vi "Project.vi"() -> ()   [LabVIEW 2022 SP3]
uses:
  Control 3.ctl
  Control 1.ctl
  <vilib>/numeric/Random Number (Range) U64.vi
  <vilib>/numeric/sub_Random U32.vi
panel:
  out "Solar pannels manager":T1(tab)
  in  "Slide 26":u8(slide)
  in  "Move to Next State":bool
  out "Discharge State":bool
  out "Charging State":bool
  in  "State selector":bool
  out "summer":picture
  out "spring":picture
  out "winter":picture
  out "Fall":picture
  out "2D Picture":picture
  out "The project is recomended":bool
  out "CRT meter 2":dbl(knob) scale=0.0..10.0
  out "CRT (years) 2":dbl
  in  "Choose your season":enum16{"Winter", "Spring", "Summer", "Fall"}(ring)
  out "IRR":dbl
  in  "Interest Rate %":dbl min=0.0 max=100.0 step=1.0 format="%#_3g"
  in  "Private Generator Availability":bool
  out "Unit Cost":dbl
  out "CRT meter":dbl(knob) scale=0.0..10.0
  out "Unit Cost 2":dbl
  out "Nominal Capacity (kWh)":dbl
  in  "Battery Type":T2(ring)
  out "Min":dbl
  out "Max":dbl
  out "DOD":dbl
  out "Efficiency 2":dbl
  out "Battery capacity (Ah)":dbl
  out "Nominal voltage":dbl
  out "Properties 2":string
  out "Conventional CRT (years)":dbl
  out "Yearly Saving ($)":dbl
  out "Total Installation Cost($)":dbl
  out "BOM($)":dbl
  in  "kWh price ($/kWh)":dbl min=0.0 step=0.01
  out "Numbers of Batteries":dbl
  out "Battery & Inverter Compatibility":string
  out "Number of series (BAT)":dbl
  out "Required Number of Panels":dbl
  in  "Location index":dbl(slide)=5.0 min=4.0 max=8.0 step=1.0 scale=4.0..8.0 scale format="%#_1g"
  out "Reqired Daily Production":dbl
  out "Required Pack Capacity":dbl
  out "Average Consuption":dbl
  in  "Minimum Backup Time (hour)":dbl=6.0 min=6.0 max=24.0 step=1.0 format="%#_2g"
  in  "Monthly Energy Consumption":dbl min=0.0
  in  "Safety factor":dbl=1.25 min=1.25 max=2.0 step=0.01 format="%#_3g"
  out "Total System maximum Draw":dbl
  out "Battery Pack Voltage":dbl
  out "Inverter efficiency":dbl
  out "RMS per phase voltage":dbl
  out "Rated Output Power (kW/PP)":dbl
  out "Triphase":bool
  out "Monophase":bool
  in  "Three-phase-system":bool
  out "Max 2":dbl format="%#_2g"
  in  "Max load ( per phase in kW)":dbl(slide) min=0.0 step=1.0 scale=0.0..50.0 scale format="%#_2g"
  out "INVERTER RECOMANDATION":string
  in  "Solar Panel Type":T3(ring)
  out "Efficiency":dbl
  out "Cost per panel":dbl
  out "Rated power":dbl
  out "Properties":string
  in  "Simulate Charging":bool
  in  "LOAD":dbl(slide) min=0.0 max=99.0 step=1.0 scale=0.0..100.0
  in  "Next State":bool
  in  "Seasons effect":bool
  in  "Light Intensity/ Irradiance, W/m^2:":dbl(knob)=600.0 min=0.0 max=2000.0 step=1.0 scale=0.0..1200.0
  in  "BATTERY CAPACITY (OV)":bool
  in  "Current Batterie %":dbl
  out "Batteries Power":dbl(knob) scale=0.0..10.0
  out "I_E":dbl
  out "Charge_Time":dbl
  out "BAT_DOD":dbl
  out "BAT_E":dbl
  in  "BATTERY PACK CAPACITY (OV)":dbl
  out "Array Rated power":dbl
  in  "Season":T4
  out "Solar Panel instantaneous P":dbl(knob) scale=0.0..10.0
  out "Load -Usage":dbl(knob) scale=0.0..2.0
  out "Private Generator 2":dbl(knob) scale=0.0..3.0
  out "Battery Level 2":dbl(slide) scale=0.0..100.0
  in  "Next State":bool
  in  "Start Simulation":bool
  in  "Load override":bool
  out "Batteries Power 2":dbl(knob) scale=0.0..10.0
  out "Load 3":dbl(knob) scale=0.0..5.0
  out "Private-Generatot 3":dbl(knob) scale=0.0..3.0
  out "Battery Level 3":dbl(slide) scale=0.0..100.0
  in  "Load override\n( per phase in kW)":dbl(slide) scale=0.0..10.0
  out "Total_Discharge_Time":dbl
  in  "Season 2":T4
  out "BAT_DOD 2":dbl
  out "I_E 2":dbl
  in  "Go back to Initialize":bool
  out "MESSAGE":string
  in  "Slide 25":u8(slide)
  # "SOLAR PANEL DESIGN"
  # "MADE BY"
  # "ELIAS ISHAK \nGEORGE YAMMINE \nELIE NAJM \nELIAS RIZK \nJACQUES MKHAYEL \nCHRISTOPHE RECHDAN"
  # "Economy"
  # "bekaaa"
  # "north ,south"
  # "beirut"
  # "matn"
  # "Thank You For Choosing us"
  # "About us :"
  # "About us:\nkindly check our website @ \nsolarpannelsmanager.com"
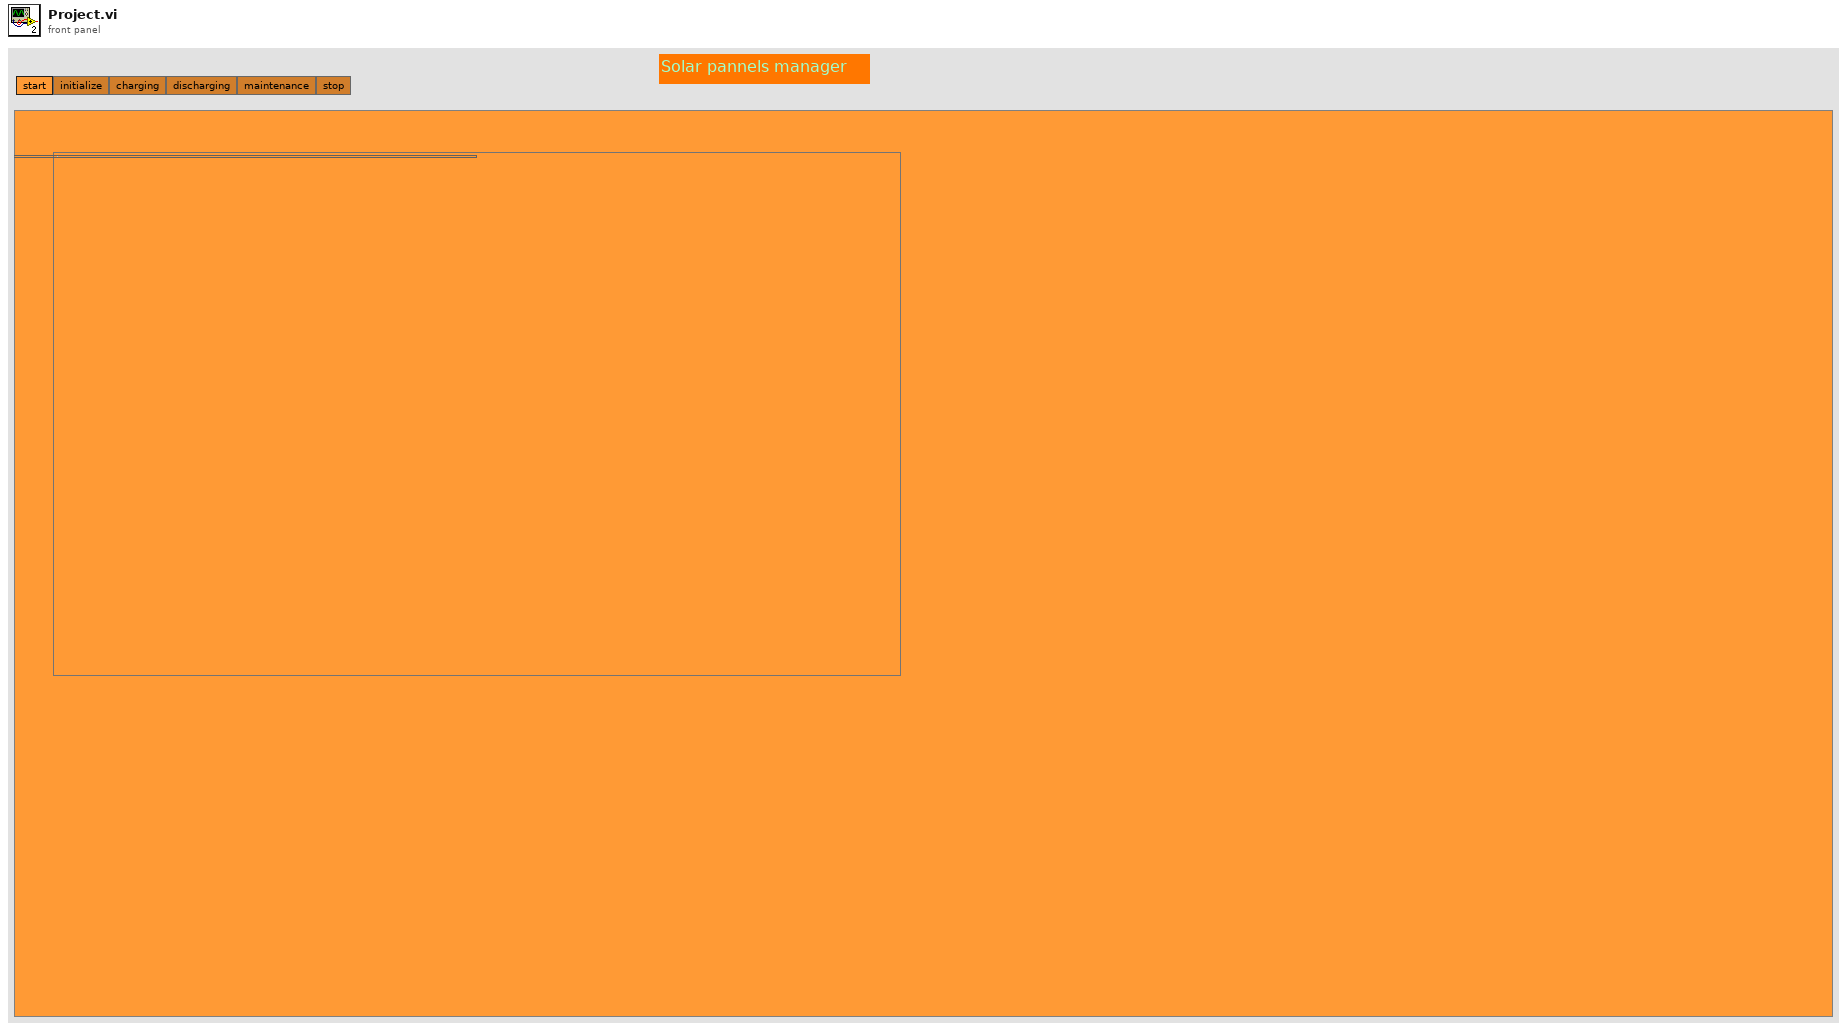
[diagram p1: front panel]
types:
  T1 = enum32{"start", "initialize", "charging", "discharging", "maintenance", "stop"}
  T2 = enum16{"Lead acid flood", "Lead acid sealed", "Lead acid agm", "Li-ion", "Li-FePO4", "Li-po"}
  T3 = enum16{"Monocrinstalin-biface", "Monocristalin", "Polycristalin", "Amorph"}
  T4 = typedef "Control 3.ctl" = enum16{"Fall", "Spring", "Winter", "Summer"}
  T5 = typedef "Control 1.ctl" = enum16{"start state ", "Initialize State", "charging state ", "discharging state ", "maintenance ", "Stop State"}
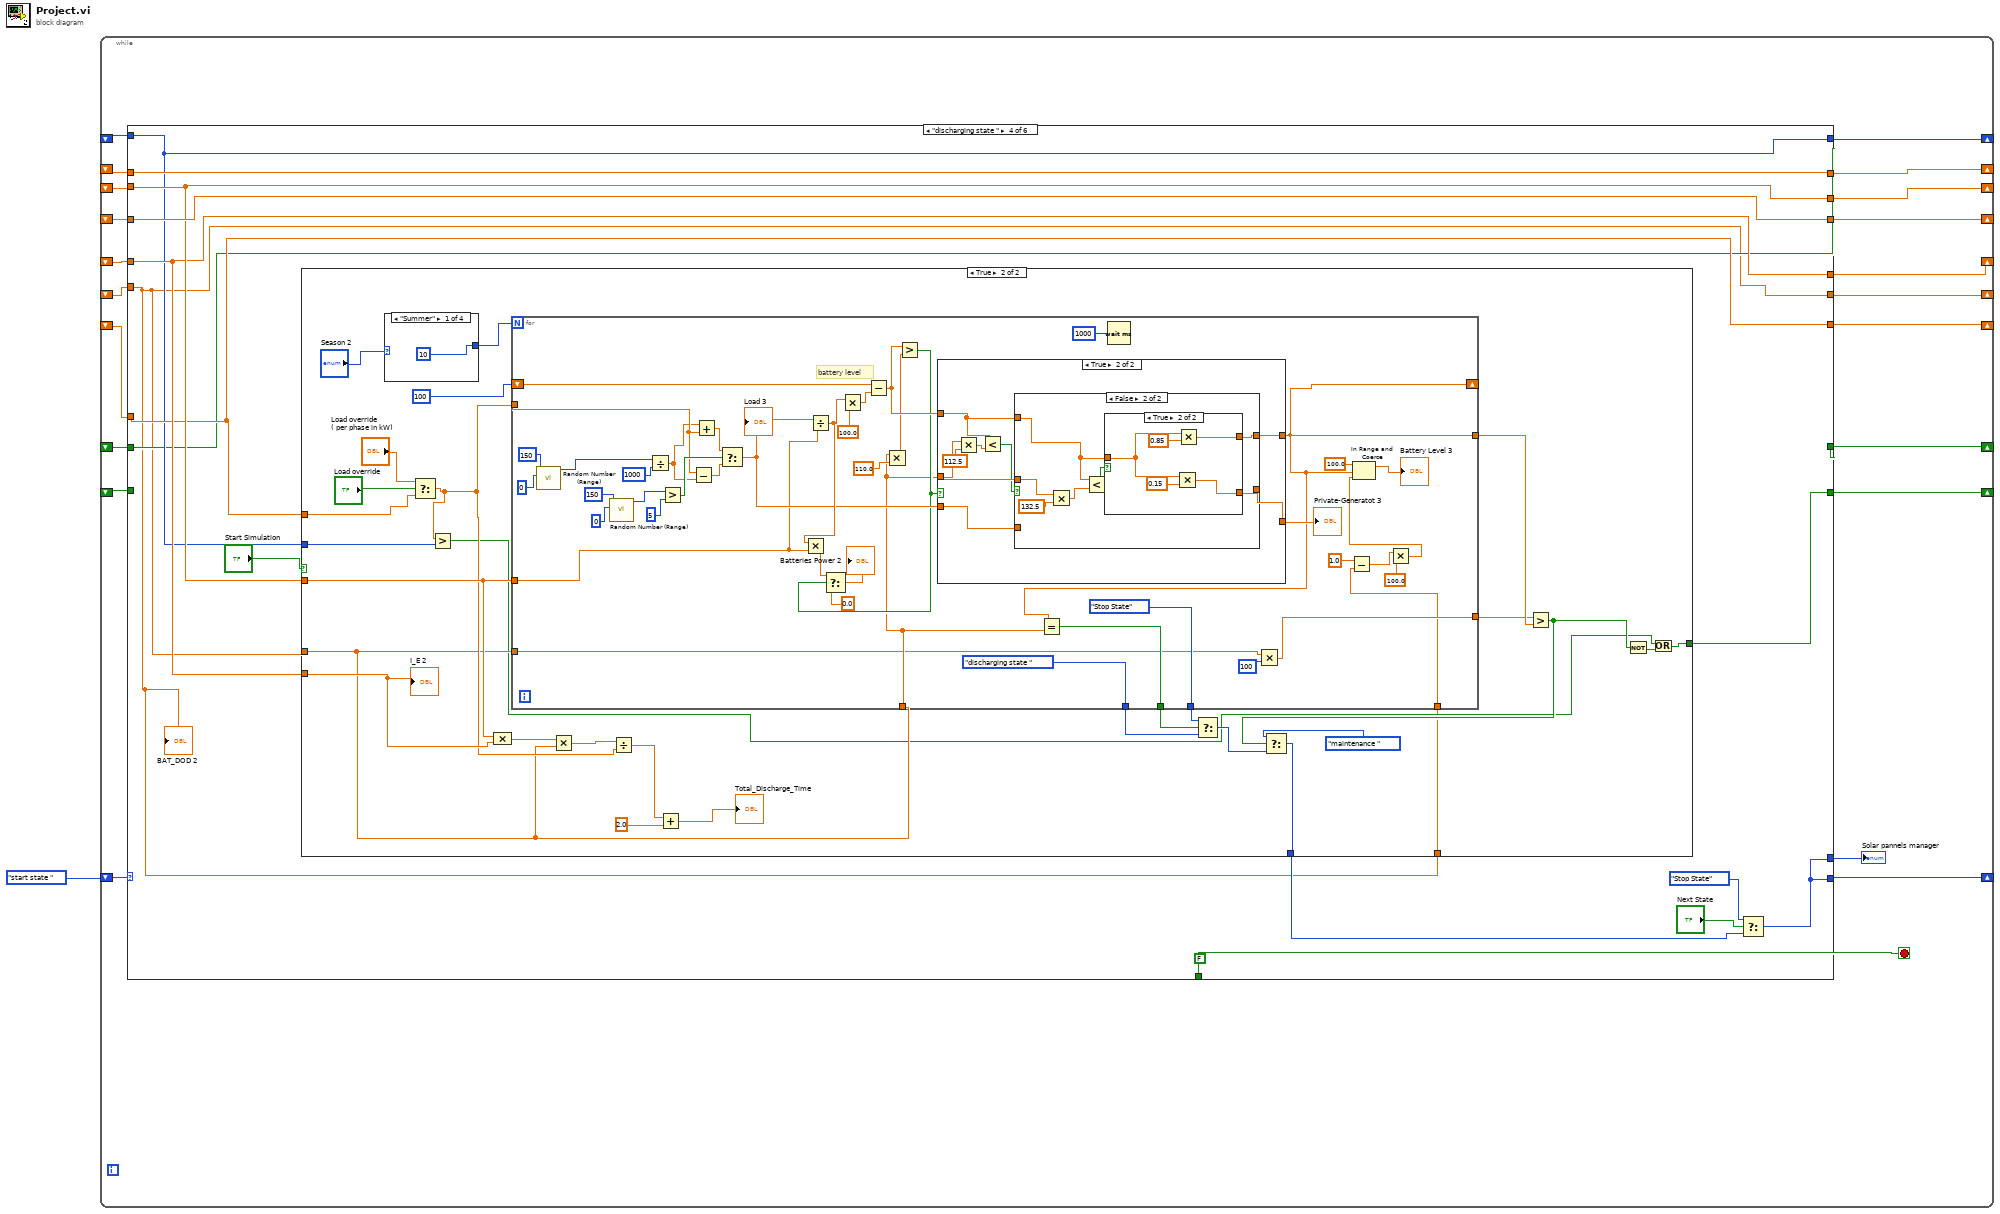
[diagram p0: block diagram]
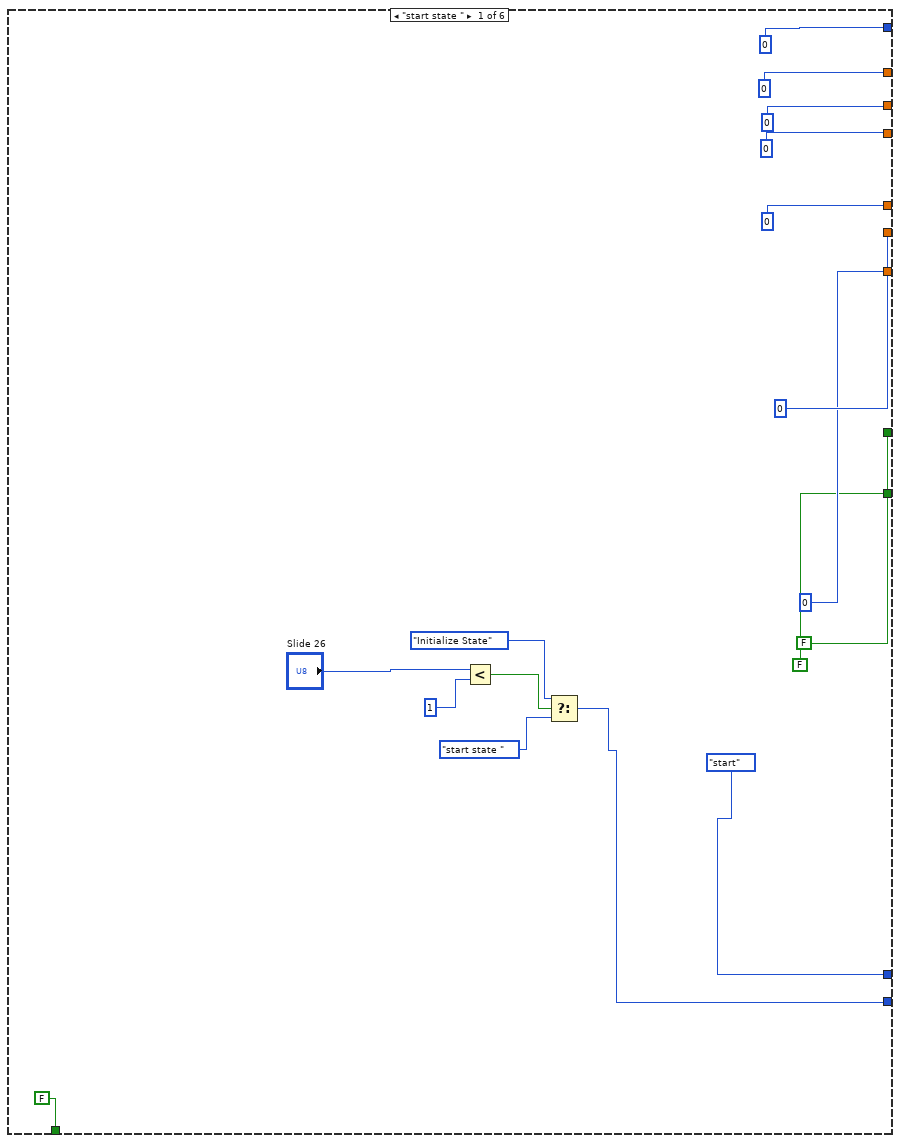
[diagram p2: hidden frame]
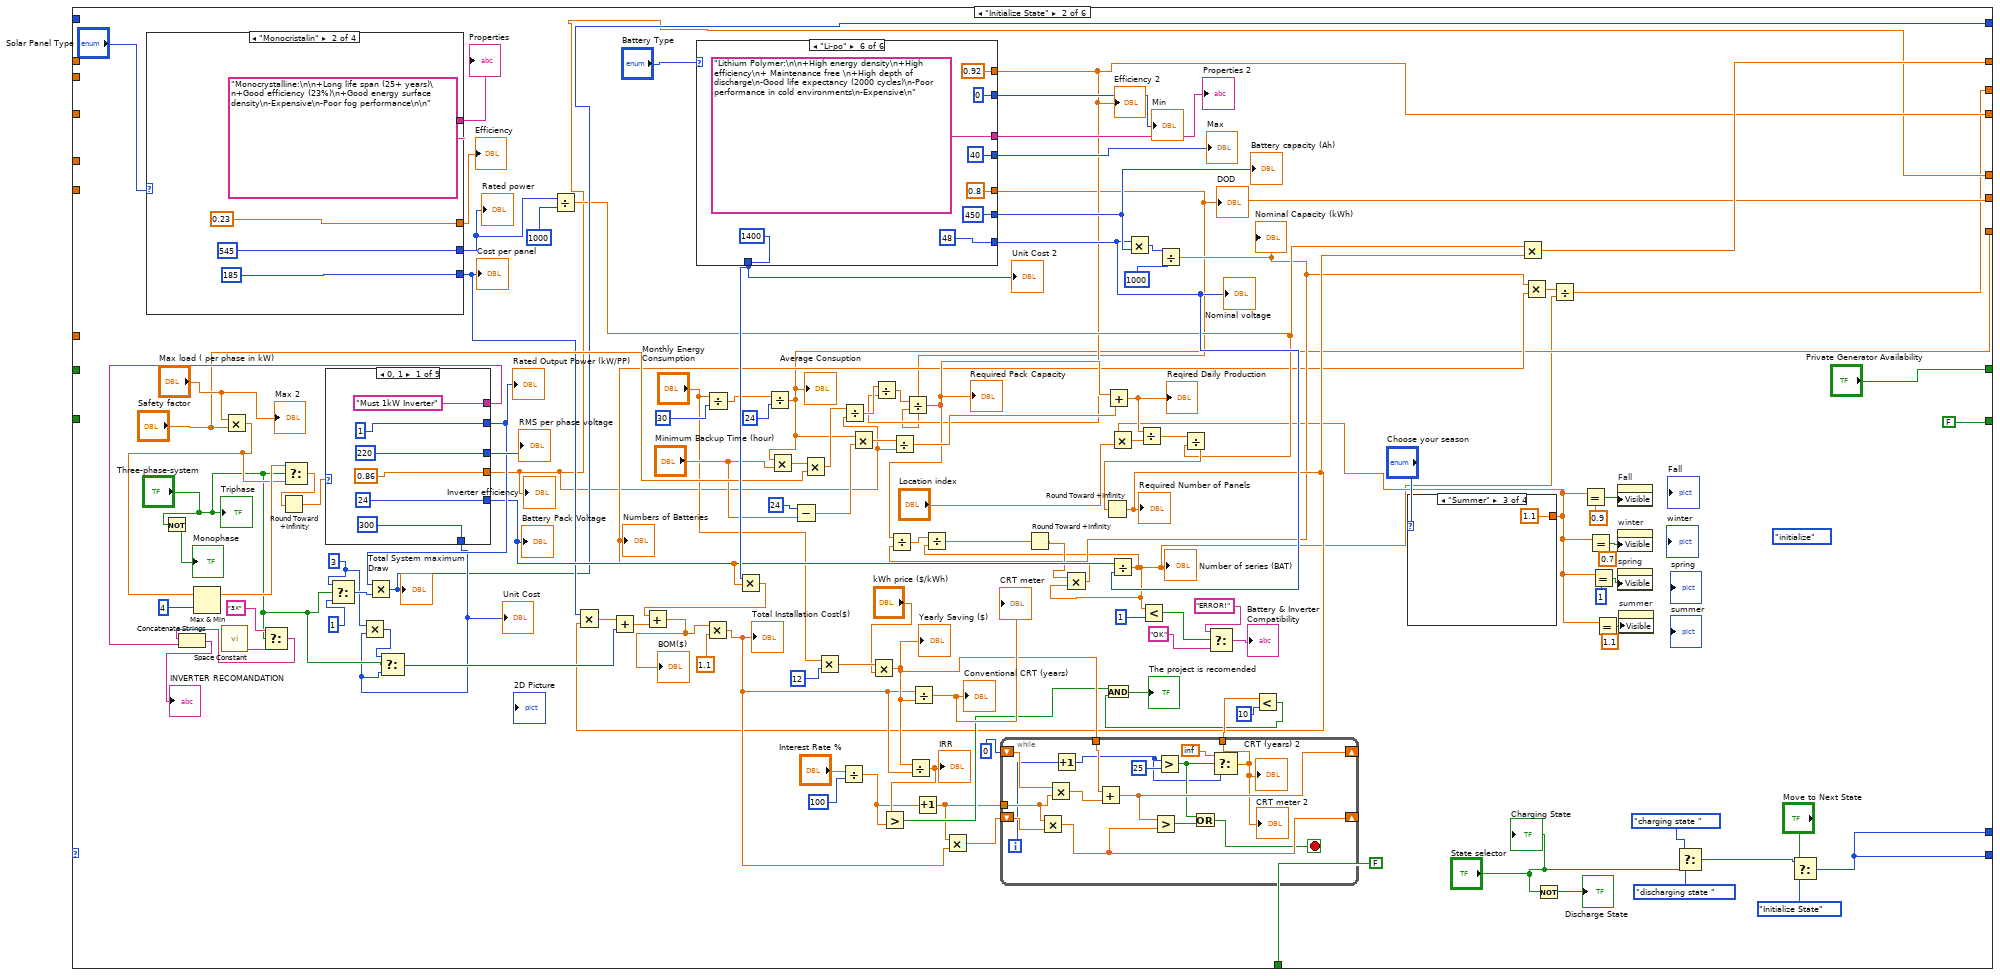
[diagram p3: hidden frame]
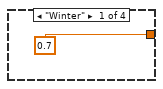
[diagram p4: hidden frame]
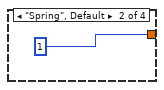
[diagram p5: hidden frame]
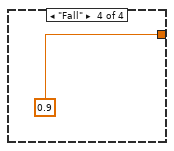
[diagram p6: hidden frame]
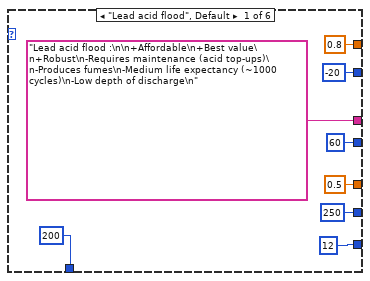
[diagram p7: hidden frame]
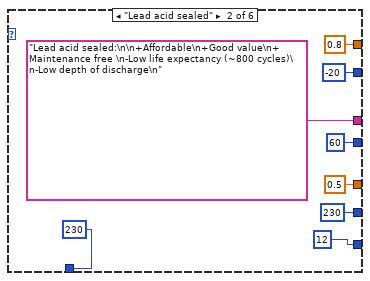
[diagram p8: hidden frame]
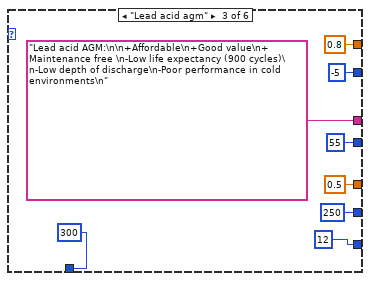
[diagram p9: hidden frame]
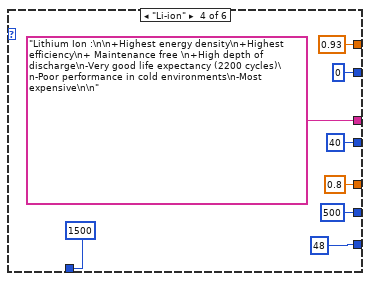
[diagram p10: hidden frame]
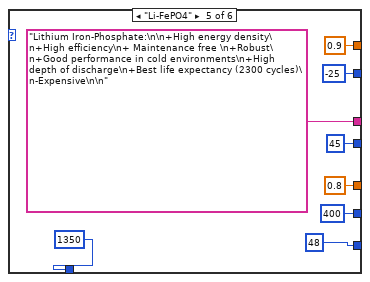
[diagram p11: hidden frame]
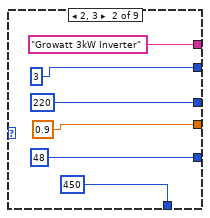
[diagram p12: hidden frame]
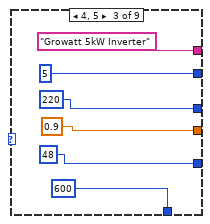
[diagram p13: hidden frame]
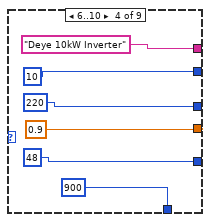
[diagram p14: hidden frame]
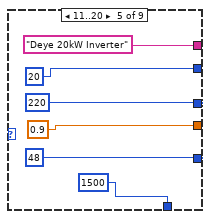
[diagram p15: hidden frame]
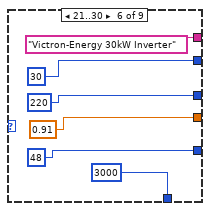
[diagram p16: hidden frame]
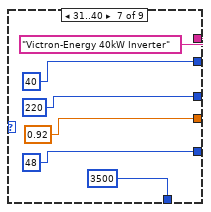
[diagram p17: hidden frame]
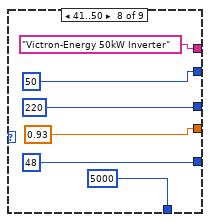
[diagram p18: hidden frame]
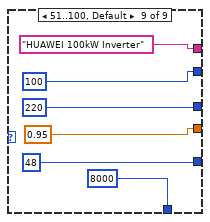
[diagram p19: hidden frame]
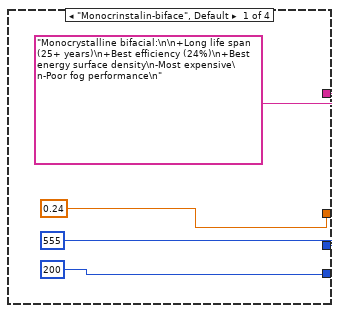
[diagram p20: hidden frame]
diagram:
  n1 = while {
    shift-right: [w22] -> _
    shift-left: Control_1."start state " ("Status") -> [w23]
    shift-right: [w19] -> _
    shift-left: _ -> [w18]
    shift-right: [w17] -> _
    shift-left: _ -> [w16]
    shift-right: [w14] -> _
    shift-left: _ -> [w15]
    shift-right: [w12] -> _
    shift-left: _ -> [w13]
    shift-right: [w10] -> _
    shift-left: _ -> [w11]
    shift-right: [w8] -> _
    shift-left: _ -> [w9]
    shift-right: [w7] -> _
    shift-left: _ -> [w6]
    shift-right: [w5] -> _
    shift-left: _ -> [w4]
    shift-right: [w2] -> _
    shift-left: _ -> [w3]
    stop <- w21 stop-if-true
    n2 = case shown="\"discharging state \"" w23 {
      tunnel: [w29 w48 w305 w434 w554 w576] -> w22
      tunnel: [FALSE FALSE FALSE FALSE FALSE TRUE] -> w21
      tunnel: [T1."start" ("Tab Control") w48 w305 w434 w554 T1."stop" ("Tab Control")] -> w20
      tunnel: [0 w58 w312 w440 w574 0] -> w19
      tunnel: w18 -> [_ _ w312 w440 w574 _]
      tunnel: [0 w55 w319 w445 w573 0] -> w17
      tunnel: w16 -> [_ _ w319 w445 w573 _]
      tunnel: w15 -> [_ _ w318 w443 w572 _]
      tunnel: [0 w41 w318 w443 w572 0] -> w14
      tunnel: w13 -> [_ _ w317 w444 w571 _]
      tunnel: [0 w52 w317 w444 w571 0] -> w12
      tunnel: w11 -> [_ _ w316 w442 w570 _]
      tunnel: [0 w51 w316 w442 w570 0] -> w10
      tunnel: w9 -> [_ _ w315 w432 w569 _]
      tunnel: [0 w50 w315 w432 w569 0] -> w8
      tunnel: [0 w47 w310 w441 w568 0] -> w7
      tunnel: w6 -> [_ _ w310 w441 w568 _]
      tunnel: [FALSE "Private Generator Availability" w309 w433 w567 FALSE] -> w5
      tunnel: w4 -> [_ _ w309 w433 w567 _]
      tunnel: [FALSE FALSE w308 w439 w564 FALSE] -> w2
      tunnel: w3 -> [_ _ _ _ w564 _]
      frame "start state " {
        n3 = Less?(x="Slide 26", y=1) -> (x < y?=w25:bool)
        n4 = Select(t=Control_1."Initialize State" ("Status"), s=w25, f=Control_1."start state " ("Status")) -> (s? t:f=w29:T5)
      }
      frame "Initialize State" {
        w113 = 3
        (unwired) T1."initialize" ("Tab Control")
        n5 = case shown="\"Monocristalin\"" "Solar Panel Type" {
          tunnel: ["Monocrystalline bifacial:\n\n+Long life span (25+ years)\n+Best efficiency (24%)\n+Best energy surface density\n-Most expensive\n-Poor fog performance\n" "Monocrystalline:\n\n+Long life span (25+ years)\n+Good efficiency (23%)\n+Good energy surface density\n-Expensive\n-Poor fog performance\n\n" "Polycrystalline:\n\n+Good life span (15+ years)\n+Offers the best value\n+Good efficiency (20%)\n-Poor fog performance\n\n" "Amorphous:\n\n+Acceptable life span (10+ years)\n+Affordable\n+Good fog performance \n-Low efficiency (10%)\n\n"] -> w160
          tunnel: [555 545 500 200] -> w98
          tunnel: [0.24 0.23 0.2 0.1] -> w159
          tunnel: [200 185 160 100] -> w96
          frame "Monocrinstalin-biface", Default {
          }
          frame "Monocristalin" {
          }
          frame "Polycristalin" {
          }
          frame "Amorph" {
          }
        }
        "Properties" <- w160
        "Rated power" <- w98
        "Cost per panel" <- w96
        "Efficiency" <- w159
        n6 = Not(x="Three-phase-system") -> (.not. x?=→"Monophase":bool)
        n7 = call <vilib>:"Space Constant.vi"() -> ("String"=w153:string)
        n8 = Multiply(x="Max load ( per phase in kW)", y="Safety factor") -> (x*y=w147:dbl)
        n9 = Max & Min(x=w147, y=4) -> (max(x,y)=w155:dbl)  [unwired: 1 out]
        n10 = Select(t="3X", s="Three-phase-system", f=w153) -> (s? t:f=w152:string)
        n11 = Select(t=w155, s="Three-phase-system", f=w147) -> (s? t:f=w105:dbl)
        n12 = Round Toward +Infinity(x=w105) -> (ceil(x): smallest int >= x=w104:dbl)
        n13 = case shown="0, 1" w104 {
          tunnel: ["Must 1kW Inverter" "Growatt 3kW Inverter" "Growatt 5kW Inverter" "Deye 10kW Inverter" "Deye 20kW Inverter" "Victron-Energy 30kW Inverter" "Victron-Energy 40kW Inverter" "Victron-Energy 50kW Inverter" "HUAWEI 100kW Inverter"] -> w151
          tunnel: [1 3 5 10 20 30 40 50 100] -> w145
          tunnel: [220 220 220 220 220 220 220 220 220] -> w149
          tunnel: [0.86 0.9 0.9 0.9 0.9 0.91 0.92 0.93 0.95] -> w51
          tunnel: [24 48 48 48 48 48 48 48 48] -> w127
          tunnel: [300 450 600 900 1500 3000 3500 5000 8000] -> w92
          frame 0, 1 {
          }
          frame 2, 3 {
          }
          frame 4, 5 {
          }
          frame 6..10 {
          }
          frame 11..20 {
          }
          frame 21..30 {
          }
          frame 31..40 {
          }
          frame 41..50 {
          }
          frame 51..100, Default {
          }
        }
        "Rated Output Power (kW/PP)" <- w145
        "RMS per phase voltage" <- w149
        "Inverter efficiency" <- w51
        "Battery Pack Voltage" <- w127
        "Unit Cost" <- w92
        n14 = Concatenate Strings(w152, w151) -> (→"INVERTER RECOMANDATION":string)
        n15 = Select(t=w113, s="Three-phase-system", f=1) -> (s? t:f=w146:i32)
        n16 = Multiply(x=w113, y=w92) -> (x*y=w114:i32)
        n17 = Multiply(x=w145, y=w146) -> (x*y=w58:i32)
        "Total System maximum Draw" <- w58
        n18 = Select(t=w114, s="Three-phase-system", f=w92) -> (s? t:f=w115:i32)
        n19 = Divide(x=w98, y=1000) -> (x/y=w57:dbl)
        n20 = case shown="\"Li-po\"" "Battery Type" {
          tunnel: ["Lead acid flood :\n\n+Affordable\n+Best value\n+Robust\n-Requires maintenance (acid top-ups)\n-Produces fumes\n-Medium life expectancy (~1000 cycles)\n-Low depth of discharge\n" "Lead acid sealed:\n\n+Affordable\n+Good value\n+ Maintenance free \n-Low life expectancy (~800 cycles)\n-Low depth of discharge\n" "Lead acid AGM:\n\n+Affordable\n+Good value\n+ Maintenance free \n-Low life expectancy (900 cycles)\n-Low depth of discharge\n-Poor performance in cold environments\n" "Lithium Ion :\n\n+Highest energy density\n+Highest efficiency\n+ Maintenance free \n+High depth of discharge\n-Very good life expectancy (2200 cycles)\n-Poor performance in cold environments\n-Most expensive\n\n" "Lithium Iron-Phosphate:\n\n+High energy density\n+High efficiency\n+ Maintenance free \n+Robust\n+Good performance in cold environments\n+High depth of discharge\n+Best life expectancy (2300 cycles)\n-Expensive\n\n" "Lithium Polymer:\n\n+High energy density\n+High efficiency\n+ Maintenance free \n+High depth of discharge\n-Good life expectancy (2000 cycles)\n-Poor performance in cold environments\n-Expensive\n"] -> w103
          tunnel: [0.5 0.5 0.5 0.8 0.8 0.8] -> w50
          tunnel: [0.8 0.8 0.8 0.93 0.9 0.92] -> w52
          tunnel: [12 12 12 48 48 48] -> w82
          tunnel: [250 230 250 500 400 450] -> w99
          tunnel: [60 60 55 40 45 40] -> w102
          tunnel: [-20 -20 -5 0 -25 0] -> w101
          tunnel: [200 230 300 1500 1350 1400] -> w161
          frame "Lead acid flood", Default {
          }
          frame "Lead acid sealed" {
          }
          frame "Lead acid agm" {
          }
          frame "Li-ion" {
          }
          frame "Li-FePO4" {
          }
          frame "Li-po" {
          }
        }
        "Properties 2" <- w103
        "Nominal voltage" <- w82
        "Battery capacity (Ah)" <- w99
        "Efficiency 2" <- w52
        "DOD" <- w50
        "Max" <- w102
        "Min" <- w101
        "Unit Cost 2" <- w161
        n21 = Divide(x="Monthly Energy Consumption", y=30) -> (x/y=w138:dbl)
        n22 = Divide(x=w138, y=24) -> (x/y=w47:dbl)
        "Average Consuption" <- w47
        n23 = Multiply(x=w47, y="Minimum Backup Time (hour)") -> (x*y=w140:dbl)
        n24 = Subtract(x=24, y="Minimum Backup Time (hour)") -> (x-y=w133:dbl)
        n25 = Multiply(x=w140, y="Safety factor") -> (x*y=w135:dbl)
        n26 = Multiply(x="Monthly Energy Consumption", y=12) -> (x*y=w107:dbl)
        n27 = Divide(x="Interest Rate %", y=100) -> (x/y=w87:dbl)
        n28 = Divide(x=w135, y=w51) -> (x/y=w136:dbl)
        n29 = Multiply(x=w47, y=w133) -> (x*y=w137:dbl)
        n30 = Multiply(x=w107, y="kWh price ($/kWh)") -> (x*y=w86:dbl)
        "Yearly Saving ($)" <- w86
        n31 = Divide(x=w136, y=w52) -> (x/y=w141:dbl)
        n32 = Divide(x=w137, y=w51) -> (x/y=w134:dbl)
        n33 = Divide(x=w141, y=w50) -> (x/y=w121:dbl)
        "Required Pack Capacity" <- w121
        n34 = Increment(x=w87) -> (x+1=w75:dbl)
        n35 = Add(x=w121, y=w134) -> (x+y=w130:dbl)
        "Reqired Daily Production" <- w130
        n36 = Divide(x=w127, y=w82) -> (x/y=w42:dbl)
        "Number of series (BAT)" <- w42
        n37 = Multiply(x=w82, y=w99) -> (x*y=w94:i32)
        n38 = Less?(x=w42, y=1) -> (x < y?=w125:bool)
        n39 = Divide(x=w94, y=1000) -> (x/y=w54:dbl)
        "Nominal Capacity (kWh)" <- w54
        n40 = Divide(x=w121, y=w54) -> (x/y=w120:dbl)
        n41 = Divide(x=w120, y=w42) -> (x/y=w119:dbl)
        n42 = Round Toward +Infinity(x=w119) -> (ceil(x): smallest int >= x=w118:dbl)
        n43 = Multiply(x=w118, y=w42) -> (x*y=w53:dbl)
        "Numbers of Batteries" <- w53
        n44 = Multiply(x=w161, y=w53) -> (x*y=w111:dbl)
        n45 = Select(t="ERROR!", s=w125, f="OK") -> (s? t:f=→"Battery & Inverter Compatibility":string)
        n46 = case shown="\"Summer\"" "Choose your season" {
          tunnel: [0.7 1 1.1 0.9] -> w44
          frame "Winter" {
          }
          frame "Spring", Default {
          }
          frame "Summer" {
          }
          frame "Fall" {
          }
        }
        n47 = Multiply(x=w44, y="Location index") -> (x*y=w84:dbl)
        n48 = Divide(x=w130, y=w84) -> (x/y=w129:dbl)
        n49 = Divide(x=w129, y=w57) -> (x/y=w128:dbl)
        n50 = Round Toward +Infinity(x=w128) -> (ceil(x): smallest int >= x=w56:dbl)
        "Required Number of Panels" <- w56
        n51 = Multiply(x=w96, y=w56) -> (x*y=w117:dbl)
        n52 = Add(x=w117, y=w115) -> (x+y=w112:dbl)
        n53 = Add(x=w111, y=w112) -> (x+y=w109:dbl)
        "BOM($)" <- w109
        n54 = Multiply(x=w109, y=1.1) -> (x*y=w74:dbl)
        "Total Installation Cost($)" <- w74
        n55 = Divide(x=w86, y=w74) -> (x/y=w88:dbl)
        "IRR" <- w88
        n56 = Greater?(x=w88, y=w87) -> (0:w76:bool)
        n57 = Divide(x=w74, y=w86) -> (x/y=→"Conventional CRT (years)" →"CRT meter":dbl)
        n58 = Multiply(x=w75, y=w74) -> (x*y=w73:dbl)
        n59 = while {
          shift-right: [w180] -> _
          shift-left: 0 -> [w178]
          tunnel: w86 -> [w177]
          shift-right: [w179] -> _
          shift-left: w73 -> [w181]
          tunnel: [w170] -> w78
          tunnel: w75 -> [w169]
          i -> [w167]
          stop <- w172 stop-if-true
          n60 = Multiply(x=w169, y=w181) -> (x*y=w179:dbl)
          n61 = Multiply(x=w178, y=w169) -> (x*y=w176:dbl)
          n62 = Increment(x=w167) -> (x+1=w168:i32)
          n63 = Add(x=w177, y=w176) -> (x+y=w180:dbl)
          n64 = Greater?(x=w180, y=w179) -> (0:w173:bool)
          n65 = Greater?(x=w168, y=25) -> (0:w171:bool)
          n66 = Or(x=w171, y=w173) -> (x .or. y?=w172:bool)
          n67 = Select(t=inf, s=w171, f=w168) -> (s? t:f=w170:dbl)
          "CRT (years) 2" <- w170
          "CRT meter 2" <- w170
        }
        n68 = Less?(x=w78, y=10) -> (x < y?=w77:bool)
        n69 = And(x=w76, y=w77) -> (x .and. y?=→"The project is recomended":bool)
        n70 = Multiply(x=w57, y=w56) -> (x*y=w55:dbl)
        n71 = Multiply(x=w54, y=w53) -> (x*y=w43:dbl)
        n72 = Not(x="State selector") -> (.not. x?=→"Discharge State":bool)
        n73 = Divide(x=w43, y=w42) -> (x/y=w41:dbl)
        n74 = Equal?(x=w44, y=0.9) -> (x = y?=w71:bool)
        n75 = Equal?(x=w44, y=0.7) -> (x = y?=w69:bool)
        n76 = Equal?(x=w44, y=1) -> (x = y?=w67:bool)
        n77 = Equal?(x=w44, y=1.1) -> (x = y?=w65:bool)
        n78 = property on="Fall" class="Pict"("Visible"=w71) -> ()  [unwired: 2 in, 2 out]
        n79 = property on="winter" class="Pict"("Visible"=w69) -> ()  [unwired: 2 in, 2 out]
        n80 = property on="spring" class="Pict"("Visible"=w67) -> ()  [unwired: 2 in, 2 out]
        n81 = property on="summer" class="Pict"("Visible"=w65) -> ()  [unwired: 2 in, 2 out]
        n82 = Select(t=Control_1."charging state " ("Status"), s="State selector", f=Control_1."discharging state " ("Status")) -> (s? t:f=w62:T5)
        n83 = Select(t=w62, s="Move to Next State", f=Control_1."Initialize State" ("Status")) -> (s? t:f=w48:T5)
        "Max 2" <- "Max load ( per phase in kW)"
        "Triphase" <- "Three-phase-system"
        "Charging State" <- "State selector"
      }
      frame "charging state " {
        w306 = Control_1."maintenance " ("Status")
        n84 = Greater?(x="LOAD", y=w312) -> (0:w302:bool)
        n85 = case shown="True" "Simulate Charging" {
          tunnel: "LOAD" -> [w338 _]
          tunnel: w319 -> [w321 _]
          tunnel: w318 -> [w334 _]
          tunnel: w317 -> [w333 _]
          tunnel: w316 -> [w332 _]
          tunnel: w315 -> [w331 _]
          tunnel: [TRUE FALSE] -> w308
          tunnel: w302 -> [w324 _]
          tunnel: [w323 Control_1."charging state " ("Status")] -> w301
          frame True {
            n86 = Divide(x="Light Intensity/ Irradiance, W/m^2:", y=1000) -> (x/y=w328:dbl)
            n87 = Select(t=w334, s="BATTERY CAPACITY (OV)", f="BATTERY PACK CAPACITY (OV)") -> (s? t:f=w336:dbl)
            n88 = Multiply(x=w328, y=w321) -> (x*y=w327:dbl)
            n89 = Compound Arithmetic op=MULTIPLY(w321, w333, w332, w331) -> (w345:dbl)
            n90 = Divide(x=w336, y=w345) -> (x/y=→"Charge_Time":dbl)
            n91 = case shown="\"Fall\"" "Season" {
              tunnel: w321 -> [w407 w414 w421 w428]
              tunnel: [14 11 10 13] -> w344
              tunnel: [w404 w412 w418 w426] -> w343
              tunnel: w327 -> [w403 w409 w417 w423]
              tunnel: "Seasons effect" -> [w405 w411 w419 w425]
              frame "Summer" {
                n92 = Multiply(x=w407, y=1.0) -> (x*y=w402:dbl)
                n93 = Select(t=w403, s=w405, f=w402) -> (s? t:f=w404:dbl)
              }
              frame "Fall" {
                n94 = Multiply(x=w414, y=0.5) -> (x*y=w410:dbl)
                n95 = Select(t=w409, s=w411, f=w410) -> (s? t:f=w412:dbl)
              }
              frame "Winter" {
                n96 = Multiply(x=w421, y=0.35) -> (x*y=w416:dbl)
                n97 = Select(t=w417, s=w419, f=w416) -> (s? t:f=w418:dbl)
              }
              frame "Spring" {
                n98 = Multiply(x=w428, y=0.7) -> (x*y=w424:dbl)
                n99 = Select(t=w423, s=w425, f=w424) -> (s? t:f=w426:dbl)
              }
            }
            n100 = for {
              N: w344 -> [_]
              tunnel: w343 -> [w360]
              tunnel: w338 -> [w382]
              tunnel: w336 -> [w347]
              shift-right: [w348] -> _
              shift-left: "Current Batterie %" -> [w373]
              n101 = call-poly <vilib>:"Random Number (Range).vi"("lower bound (0)"=u64 0, "upper bound (100)"=u64 10) -> ("number"=w367:u64)  [unwired: 9 in]
              n102 = call-poly <vilib>:"Random Number (Range).vi"("lower bound (0)"=u64 0, "upper bound (100)"=u64 150) -> ("number"=w362:u64)  [unwired: 9 in]
              n103 = call-poly <vilib>:"Random Number (Range).vi"("lower bound (0)"=u64 0, "upper bound (100)"=u64 100) -> ("number"=w389:u64)  [unwired: 9 in]
              n104 = call-poly <vilib>:"Random Number (Range).vi"("lower bound (0)"=u64 0, "upper bound (100)"=u64 10) -> ("number"=w393:u64)  [unwired: 9 in]
              n105 = Divide(x=w362, y=1000.0) -> (x/y=w361:dbl)
              n106 = Greater?(x=w367, y=u64 5) -> (0:w365:bool)
              n107 = Divide(x=w389, y=u64 1000) -> (x/y=w381:dbl)
              n108 = Greater?(x=w393, y=u64 5) -> (0:w392:bool)
              n109 = Add(x=w361, y=w360) -> (x+y=w364:dbl)
              n110 = Subtract(x=w360, y=w361) -> (x-y=w363:dbl)
              n111 = Subtract(x=w382, y=w381) -> (x-y=w390:dbl)
              n112 = Add(x=w381, y=w382) -> (x+y=w391:dbl)
              n113 = Select(t=w364, s=w365, f=w363) -> (s? t:f=w355:dbl)
              "Solar Panel instantaneous P" <- w355
              n114 = Select(t=w391, s=w392, f=w390) -> (s? t:f=w375:dbl)
              "Load -Usage" <- w375
              n115 = Divide(x=w355, y=4.0) -> (x/y=w374:dbl)
              n116 = Subtract(x=w355, y=w375) -> (x-y=w401:dbl)
              n117 = Divide(x=w374, y=w347) -> (x/y=w359:dbl)
              n118 = Divide(x=w401, y=w347) -> (x/y=w358:dbl)
              n119 = Multiply(x=0.75, y=w355) -> (x*y=w356:dbl)
              n120 = Subtract(x=w375, y=w356) -> (x-y=w379:dbl)
              n121 = Multiply(x=w358, y=100.0) -> (x*y=w398:dbl)
              n122 = In Range and Coerce(upper limit=100.0, x=w379, lower limit=0.0) -> (coerced(x)=w352:dbl)  [unwired: 1 out]
              n123 = Less?(x=w398, y=0.0) -> (x < y?=w351:bool)
              n124 = Select(t=w359, s=w351, f=w358) -> (s? t:f=w357:dbl)
              n125 = Select(t=w352, s=w351, f=0.0) -> (s? t:f=w349:dbl)
              "Private Generator 2" <- w349
              n126 = Multiply(x=w347, y=w357) -> (x*y=→"Batteries Power":dbl)
              n127 = Add(x=w349, y=w373) -> (x+y=w396:dbl)
              n128 = Add(x=w373, y=w398) -> (x+y=w395:dbl)
              n129 = Select(t=w396, s=w351, f=w395) -> (s? t:f=w348:dbl)
              n130 = In Range and Coerce(upper limit=100.0, x=w348, lower limit=0.0) -> (coerced(x)=→"Battery Level 2":dbl)  [unwired: 1 out]
              n131 = Wait (ms)(milliseconds to wait=u32 1000) -> ()  [unwired: 1 out]
            }
            n132 = Select(t=Control_1."maintenance " ("Status"), s=w324, f=Control_1."discharging state " ("Status")) -> (s? t:f=w323:T5)
            "Array Rated power" <- w321
            "BAT_E" <- w333
            "BAT_DOD" <- w331
            "I_E" <- w332
          }
          frame False {
          }
        }
        n133 = Select(t=Control_1."discharging state " ("Status"), s="Next State", f=Control_1."charging state " ("Status")) -> (s? t:f=w304:T5)
        n134 = Equal?(x=w301, y=w306) -> (x = y?=w307:bool)
        n135 = Select(t=w306, s=w307, f=w304) -> (s? t:f=w305:T5)
      }
      frame "discharging state " {
        n136 = case shown="True" "Start Simulation" {
          tunnel: w443 -> [_ w467]
          tunnel: w442 -> [_ w466]
          tunnel: w441 -> [_ w462]
          tunnel: w440 -> [_ w458]
          tunnel: w432 -> [_ w457]
          tunnel: [FALSE w451] -> w439
          tunnel: [Control_1."discharging state " ("Status") w450] -> w436
          tunnel: w432 -> [_ w449]
          frame False {
          }
          frame True {
            n137 = case shown="\"Summer\"" "Season 2" {
              tunnel: [10 13 14 11] -> w476
              frame "Summer" {
              }
              frame "Fall" {
              }
              frame "Winter" {
              }
              frame "Spring" {
              }
            }
            n138 = Select(t="Load override\n( per phase in kW)", s="Load override", f=w462) -> (s? t:f=w459:dbl)
            n139 = Greater?(x=w459, y=w458) -> (0:w452:bool)
            n140 = Compound Arithmetic op=MULTIPLY(w467, w466) -> (w468:dbl)
            n141 = for {
              N: w476 -> [_]
              tunnel: w459 -> [w508]
              shift-right: [w485] -> _
              shift-left: 100 -> [w506]
              tunnel: w457 -> [w493]
              tunnel: [Control_1."discharging state " ("Status")] -> w473
              tunnel: [w492] -> w472
              tunnel: [Control_1."Stop State" ("Status")] -> w471
              tunnel: w467 -> [w489]
              tunnel: w457 -> [w488]
              tunnel: [w485] -> w456
              tunnel: [w486] -> w455
              tunnel: w449 -> [w481]
              # "battery level"
              n142 = call-poly <vilib>:"Random Number (Range).vi"("lower bound (0)"=u64 0, "upper bound (100)"=u64 150) -> ("number"=w514:u64)  [unwired: 9 in]
              n143 = call-poly <vilib>:"Random Number (Range).vi"("lower bound (0)"=u64 0, "upper bound (100)"=u64 150) -> ("number"=w518:u64)  [unwired: 9 in]
              n144 = Divide(x=w514, y=u64 1000) -> (x/y=w507:dbl)
              n145 = Greater?(x=w518, y=u64 5) -> (0:w517:bool)
              n146 = Subtract(x=w508, y=w507) -> (x-y=w515:dbl)
              n147 = Add(x=w507, y=w508) -> (x+y=w516:dbl)
              n148 = Select(t=w516, s=w517, f=w515) -> (s? t:f=w499:dbl)
              "Load 3" <- w499
              n149 = Divide(x=w499, y=w489) -> (x/y=w504:dbl)
              n150 = Multiply(x=w504, y=w489) -> (x*y=w503:dbl)
              n151 = Multiply(x=w504, y=100.0) -> (x*y=w505:dbl)
              n152 = Subtract(x=w506, y=w505) -> (x-y=w498:dbl)
              n153 = Multiply(x=w493, y=110.0) -> (x*y=w496:dbl)
              n154 = Greater?(x=w498, y=w496) -> (0:w494:bool)
              n155 = Select(t=w503, s=w494, f=0.0) -> (s? t:f=→"Batteries Power 2":dbl)
              n156 = case shown="True" w494 {
                tunnel: w498 -> [_ w525]
                tunnel: w493 -> [w522 w526]
                tunnel: [w521 w528] -> w500
                tunnel: [w522 w527] -> w485
                tunnel: w499 -> [w521 w529]
                frame False {
                }
                frame True {
                  n157 = Multiply(x=w526, y=112.5) -> (x*y=w530:dbl)
                  n158 = Less?(x=w525, y=w530) -> (x < y?=w524:bool)
                  n159 = case shown="False" w524 {
                    tunnel: w529 -> [w533 _]
                    tunnel: [w534 w536] -> w528
                    tunnel: [w531 w537] -> w527
                    tunnel: w526 -> [_ w540]
                    tunnel: w525 -> [_ w538]
                    frame True {
                      n160 = Multiply(x=w533, y=0.4) -> (x*y=w531:dbl)
                      n161 = Multiply(x=w533, y=0.6) -> (x*y=w534:dbl)
                    }
                    frame False {
                      n162 = Multiply(x=w540, y=132.5) -> (x*y=w541:dbl)
                      n163 = Less?(x=w538, y=w541) -> (x < y?=w539:bool)
                      n164 = case shown="True" w539 {
                        tunnel: w538 -> [w544 w547]
                        tunnel: [w544 w546] -> w537
                        tunnel: [0.0 w545] -> w536
                        frame False {
                        }
                        frame True {
                          n165 = Multiply(x=w547, y=0.15) -> (x*y=w545:dbl)
                          n166 = Multiply(x=w547, y=0.85) -> (x*y=w546:dbl)
                        }
                      }
                    }
                  }
                }
              }
              "Private-Generatot 3" <- w500
              n167 = Equal?(x=w493, y=w485) -> (x = y?=w492:bool)
              n168 = Wait (ms)(milliseconds to wait=u32 1000) -> ()  [unwired: 1 out]
              n169 = Multiply(x=w488, y=100) -> (x*y=w486:dbl)
              n170 = Subtract(x=1.0, y=w481) -> (x-y=w480:dbl)
              n171 = Multiply(x=w480, y=100.0) -> (x*y=w478:dbl)
              n172 = In Range and Coerce(upper limit=100.0, x=w485, lower limit=w478) -> (coerced(x)=→"Battery Level 3":dbl)  [unwired: 1 out]
            }
            n173 = Multiply(x=w468, y=w457) -> (x*y=w465:dbl)
            n174 = Divide(x=w465, y=w459) -> (x/y=w464:dbl)
            n175 = Add(x=w464, y=2.0) -> (x+y=→"Total_Discharge_Time":dbl)
            n176 = Select(t=w471, s=w472, f=w473) -> (s? t:f=w470:T5)
            n177 = Greater?(x=w455, y=w456) -> (0:w454:bool)
            n178 = Select(t=Control_1."maintenance " ("Status"), s=w454, f=w470) -> (s? t:f=w450:T5)
            n179 = Not(x=w454) -> (.not. x?=w453:bool)
            n180 = Or(x=w452, y=w453) -> (x .or. y?=w451:bool)
            "I_E 2" <- w466
          }
        }
        n181 = Select(t=Control_1."Stop State" ("Status"), s="Next State", f=w436) -> (s? t:f=w434:T5)
        "BAT_DOD 2" <- w432
      }
      frame "maintenance " {
        n182 = call <vilib>:"Space Constant.vi"() -> ("String"=w565:string)
        n183 = Select(t="SWITCHING TO PRIVATE GENERATOR ", s=w567, f=w565) -> (s? t:f=w560:string)
        n184 = Select(t="The load exceeded the maximum inverter rating \nThe inverter was turned off for safety reasons ", s=w564, f="LOW BATTERY !!!") -> (s? t:f=w561:string)
        n185 = call <vilib>:"Space Constant.vi"() -> ("String"=w559:string)
        n186 = Concatenate Strings(w561, w559, w560) -> (→"MESSAGE":string)
        n187 = Select(t=Control_1."Initialize State" ("Status"), s="Go back to Initialize", f=Control_1."maintenance " ("Status")) -> (s? t:f=w554:T5)
      }
      frame "Stop State" {
        n188 = Greater?(x="Slide 25", y=99.0) -> (0:w577:bool)
        n189 = Select(t=Control_1."start state " ("Status"), s=w577, f=Control_1."Stop State" ("Status")) -> (s? t:f=w576:T5)
      }
    }
    "Solar pannels manager" <- w20
  }
